vi "Keithley 27XX Finite Multi Read.vi"() -> ()   [LabVIEW 2020]
doc: "This example VI allows you to return an array of data from specifed channels.\n\nNote:\nFor front panel measurements, make sure the Input switch is in the out position(F)\nFor plug-in card measurements, make sure the Input switch is in the in poisition(R)"
uses:
  <instrlib>/Keithley 27XX/Public/Data/Read Multiple Direct.vi
  <instrlib>/Keithley 27XX/Keithley 27XX.lvlib
panel:
  in  "Serial Configuration":T1={"Baud Rate (9600)"=9600, "Flow Control (1: XON/XOFF)"=1, "Termination Char (0:CR)"=0} {"Termination Char (0:CR)" items=["CR", "LF"]; "Flow Control (1: XON/XOFF)" items=["None", "XON/XOFF", "RTS/CTS (2701 Only)", "XON/XOFF & RTS/CTS (2701 Only)"]; "Baud Rate (9600)" items=["300"=300, "600"=600, "1200"=1200, "2400"=2400, "4800"=4800, "9600"=9600, "19.2k"=19200, "38.4k (2701 Only)"=38400, "57.6k (2701 Only)"=57600, "115.2k (2701 Only)"=115200]}
  in  "Timeout (30000 milliseconds)":u32=30000
  in  "Sample Count (100)":i32=100
  out "Measurement Data":dbl[](array[numeric])
  in  "Function (0: DC Voltage)":u16(ring) items=["DC Voltage", "AC Voltage", "DC Current", "AC Current", "Resistance", "Four-Wire Resistance", "Temperature (C)", "Frequency", "Period", "Continuity"]
  in  "Channel List (101:110)":string="101:110"
  in  "VISA resource name":refnum<visa-resource-name>
  # "*For front panel measurements, make sure the Input switch is in the out position(F)*\n  For plug-in card measurements, make sure the Input switch is in the in position(R)"
  # "© 2005 National Instruments Corporation.  ALL RIGHTS RESERVED."
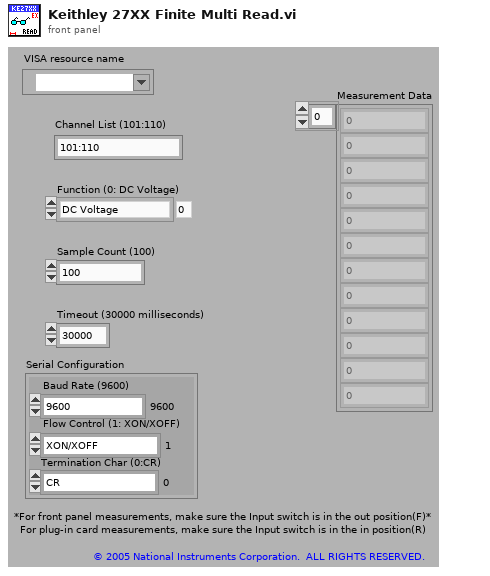
[diagram p1: front panel]
types:
  T1 = cluster{"Baud Rate (9600)":u32, "Flow Control (1: XON/XOFF)":u16, "Termination Char (0:CR)":u16}
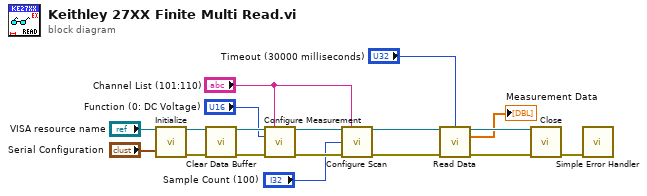
[diagram p0: block diagram]
diagram:
  n1 = call <instrlib>:"Initialize.vi"("VISA resource name"="VISA resource name", "Serial Configuration"="Serial Configuration") -> ("VISA resource name out"=w9:refnum<visa-resource-name>, "error out"=w10:errorcluster)  [unwired: 12 in]
  n2 = call <instrlib>:"Clear Data Buffer.vi"("VISA resource name"=w9, "error in (no error)"=w10) -> ("VISA resource name out"=w12:refnum<visa-resource-name>, "error out"=w11:errorcluster)  [unwired: 12 in]
  n3 = call <instrlib>:"Configure Measurement.vi"("VISA resource name"=w12, "Scan List (Empty)"="Channel List (101:110)", "Function (0: DC Voltage)"="Function (0: DC Voltage)", "error in (no error)"=w11) -> ("VISA resource name out"=w17:refnum<visa-resource-name>, "error out"=w14:errorcluster)  [unwired: 10 in]
  n4 = call <instrlib>:"Configure Scan.vi"("VISA resource name"=w17, "Channel List (101:110)"="Channel List (101:110)", "Sample Count (100)"="Sample Count (100)", "error in (no error)"=w14) -> ("VISA resource name out"=w6:refnum<visa-resource-name>, "error out"=w7:errorcluster)  [unwired: 10 in]
  n5 = call-poly <instrlib>:"Read Data.vi"("VISA resource name"=w6, "Timeout (30000 milliseconds)"="Timeout (30000 milliseconds)", "error in (no error)"=w7) -> ("VISA resource name out"=w16:refnum<visa-resource-name>, "Measurement Data"=→"Measurement Data":dbl[], "error out"=w15:errorcluster)  [unwired: 7 in, 3 out]
  n6 = call <instrlib>:"Close.vi"("VISA resource name"=w16, "error in (no error)"=w15) -> ("error out"=w13:errorcluster)  [unwired: 13 in]
  n7 = call <vilib>:"Simple Error Handler.vi"("error in (no error)"=w13) -> ()  [unwired: 4 in, 5 out]
